vi "DVR Read - PackageID.vi"(11 "Data Value Reference in":refnum<data-value>) -> (3 "PackageID":i32)   [LabVIEW 2021, in "Performanced XNET CAN Signal Logger.lvlib" / "Performanced XNET CAN Signal Logger.lvclass"]
uses:
  Performanced XNET CAN Signal Logger.lvclass
  Performanced XNET CAN Signal Logger.lvclass/Performanced XNET CAN Signal Logger.ctl
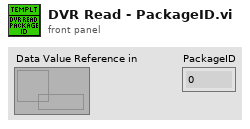
[diagram p1: front panel]
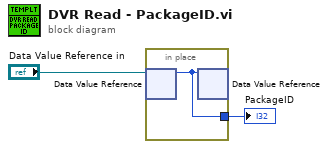
[diagram p0: block diagram]
diagram:
  n1 = in-place {
    in-place-border: [w3] -> w2
    n2 = in-place-dvr #1("Data Value Reference in") -> (w3:i32)  [unwired: 1 out]
    n3 = in-place-dvr #1(w3) -> ()  [unwired: 2 out]
  }
  "PackageID" <- w2
